vi "dfd_FXP PtByPt Lattice Allpass (normalized).vi"(6 "state in":i64[](array[numeric]), 7 "FXPOPs":T5[](array[typedef]) {"source" items=["Coef a/k"=0, "Coef b/v"=7, "Input"=1, "Output"=2, "Multiplicand"=3, "Product"=4, "Sum"=5, "Delay"=6, "Gain"=8]}, 8 "filtering statistics in":T4(array[cluster]) {"statistics information"."min value" format="%.2f"; "statistics information"."max value" format="%.2f"; "Quantizer Source" items=["Coefficients a/k"=0, "Coefficients b/v"=7, "Input"=1, "Output"=2, "Multiplicand"=3, "Product"=4, "Sum"=5, "Delay"=6]}, 9 "coef ^k[M..1]":T1, 10 "coef k[M..1]":T1, 11 "x":T7={"value"=0, "wl"=0, "iwl"=0, "Signed"=TRUE} {"value" format="%.0x"}) -> (0 "filtering statistics out":T4(array[cluster]) {"statistics information"."min value" format="%.2f"; "statistics information"."max value" format="%.2f"; "Quantizer Source" items=["Coefficients a/k"=0, "Coefficients b/v"=7, "Input"=1, "Output"=2, "Multiplicand"=3, "Product"=4, "Sum"=5, "Delay"=6]}, 3 "filtered x":T7={"value"=0, "wl"=0, "iwl"=0, "Signed"=TRUE} {"value" format="%.0x"}, 4 "state out":i64[](array[numeric]))   [LabVIEW 2017, in "NI_DigFilter_FXP.lvlib"]
uses:
  <vilib>/addons/Digital Filter Design/NI_DigFilter_FXP.lvlib
  <vilib>/addons/Digital Filter Design/_Objects.llb/dfd_DFXP Data Type (scaler).ctl
  <vilib>/addons/Digital Filter Design/_Objects.llb/dfd_DFXP Operation Parameter.ctl
  <vilib>/addons/Digital Filter Design/_Objects.llb/dfd_Internal Quantization Srcs.ctl
  <vilib>/addons/Digital Filter Design/_Objects.llb/dfd_DFXP Data Type (vector).ctl
  <vilib>/addons/Digital Filter Design/_Objects.llb/DFD Quantization Sources.ctl
  <vilib>/addons/Digital Filter Design/_Objects.llb/DFD FXP Statistics Data.ctl
  <vilib>/addons/Digital Filter Design/NI_DigFilterLicensed.lvlib
panel:
  in  "DFXP array type":T1
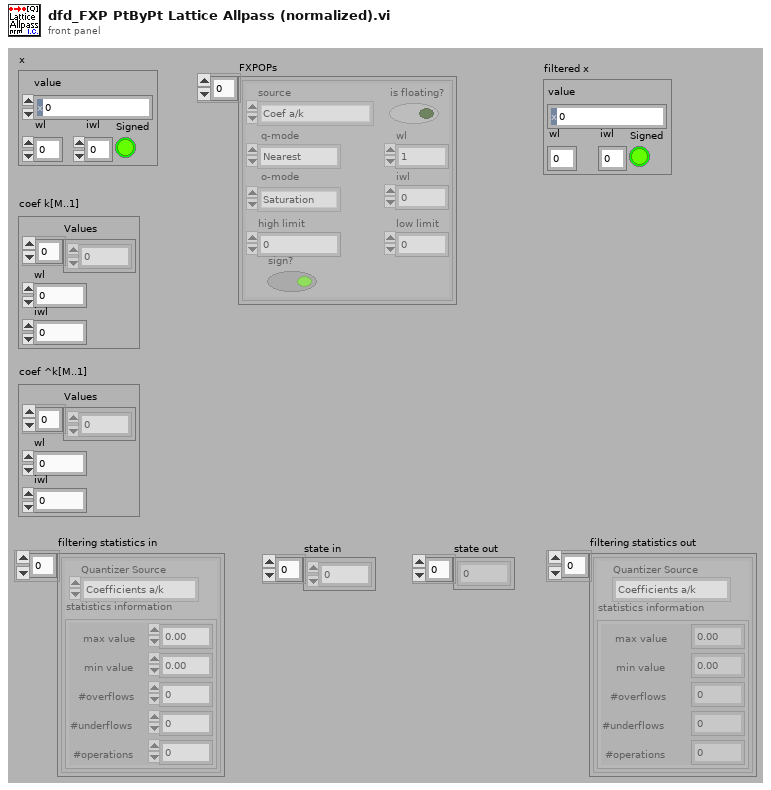
[diagram p1: front panel]
types:
  T1 = typedef "dfd_DFXP Data Type (vector).ctl" = cluster{"Values":i64[], "wl":i16, "iwl":i16}
  T2 = typedef "NI_DigFilterLicensed.lvlib/DFD Quantization Sources.ctl" = u16
  T3 = typedef "NI_DigFilterLicensed.lvlib/DFD FXP Statistics Data.ctl" = cluster{"max value":ext, "min value":ext, "#overflows":i32, "#underflows":i32, "#operations":i32}
  T4 = cluster{"Quantizer Source":T2, "statistics information":T3}[]
  T5 = typedef "dfd_DFXP Operation Parameter.ctl" = cluster{"source":T6, "is floating?":bool, "o-mode":enum16{"Saturation", "Wrap"}, "q-mode":enum16{"Nearest", "Truncation"}, "wl":i16, "high limit":i64, "low limit":i64, "iwl":i16, "sign?":bool}
  T6 = typedef "NI_DigFilterLicensed.lvlib/dfd_Internal Quantization Srcs.ctl" = u16
  T7 = typedef "dfd_DFXP Data Type (scaler).ctl" = cluster{"value":i64, "wl":i16, "iwl":i16, "Signed":bool}
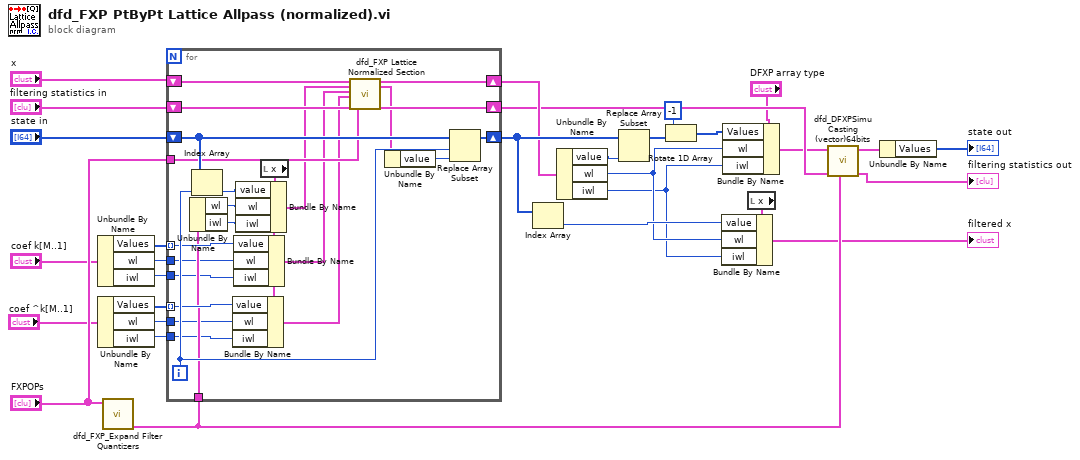
[diagram p0: block diagram]
diagram:
  n1 = Unbundle By Name("coef k[M..1]") -> ("Values"=w15:i64[], "wl"=w12:i16, "iwl"=w11:i16)
  n2 = Unbundle By Name("coef ^k[M..1]") -> ("Values"=w14:i64[], "wl"=w10:i16, "iwl"=w9:i16)
  n3 = call <vilib>:"dfd_FXP_Expand Filter Quantizers.vi"("FXPOPs"="FXPOPs") -> ("Delay"=w13:T5)  [unwired: 10 out]
  n4 = for {
    shift-right: [w51] -> w24
    shift-left: "x" -> [w52]
    shift-right: [w53] -> w25
    shift-left: "state in" -> [w54]
    tunnel: "FXPOPs" -> [w50]
    shift-right: [w47] -> w23
    shift-left: "filtering statistics in" -> [w48]
    tunnel: w15 -> [w44] mode=indexing
    tunnel: w14 -> [w43] mode=indexing
    tunnel: w13 -> [w41]
    tunnel: w12 -> [w37]
    tunnel: w11 -> [w36]
    tunnel: w10 -> [w33]
    tunnel: w9 -> [w32]
    i -> [w49]
    n5 = Unbundle By Name(w41) -> ("wl"=w40:i16, "iwl"=w39:i16)
    n6 = Index Array(array=w54, index=w49) -> (element=w45:i64)
    n7 = local read "x"() -> (w34:T7)
    n8 = Bundle By Name(cluster=w34, "value"=w43, "wl"=w33, "iwl"=w32) -> (w35:T7)
    n9 = Bundle By Name(cluster=w34, "value"=w44, "wl"=w37, "iwl"=w36) -> (w38:T7)
    n10 = Bundle By Name(cluster=w34, "value"=w45, "wl"=w40, "iwl"=w39) -> (w42:T7)
    n11 = call <vilib>:"dfd_FXP Lattice Normalized Section.vi"("x(m)"=w52, "w(m-1)"=w42, "k(m)"=w38, "^k(m)"=w35, "filtering statistics in"=w48, "FXPOPs"=w50) -> ("x(m-1)"=w51:T7, "w(m)"=w46:T7, "filtering statistics out"=w47:T4)  [unwired: 11 out]
    n12 = Unbundle By Name(w46) -> ("value"=w31:i64)
    n13 = Replace Array Subset(array=w54, new element=w31, index=w49) -> (w53:i64[])
  }
  n14 = Index Array(array=w25) -> (element=w22:i64)  [unwired: 1 in]
  n15 = Unbundle By Name(w24) -> ("value"=w8:i64, "wl"=w3:i16, "iwl"=w2:i16)
  n16 = Replace Array Subset(array=w25, new element=w8) -> (w28:i64[])  [unwired: 1 in]
  n17 = Rotate 1D Array(1:w28, 2:-1 ("n")) -> (0:w26:i64[])
  n18 = Bundle By Name(cluster="DFXP array type", "Values"=w26, "wl"=w3, "iwl"=w2) -> (w7:T1)
  n19 = local read "x"() -> (w4:T7)
  n20 = Bundle By Name(cluster=w4, "value"=w22, "wl"=w3, "iwl"=w2) -> (→"filtered x":T7)
  n21 = call <vilib>:"dfd_DFXPSimu Casting (vector)64bits.vi"("op params"=w13, "filtering statistics in"=w23, "Value in"=w7) -> ("filtering statistics out"=→"filtering statistics out":T4, "Value out"=w21:T1)  [unwired: 1 in, 6 out]
  n22 = Unbundle By Name(w21) -> ("Values"=→"state out":i64[])
